vi "Keithley 622x Set DCon.vi"(6 "Step":dbl=0.0001 format="%#_6p", 7 "Delta":dbl=0.0001 format="%#_6p", 8 "error in":errorcluster, 9 "End":dbl=0.001 format="%#_6p", 10 "Start":dbl=-0.001 format="%#_6p", 11 "VISA resource name":refnum<visa-resource-name>) -> (0 "error out":errorcluster, 3 "VISA resource name out":refnum<visa-resource-name>)   [LabVIEW 2021]
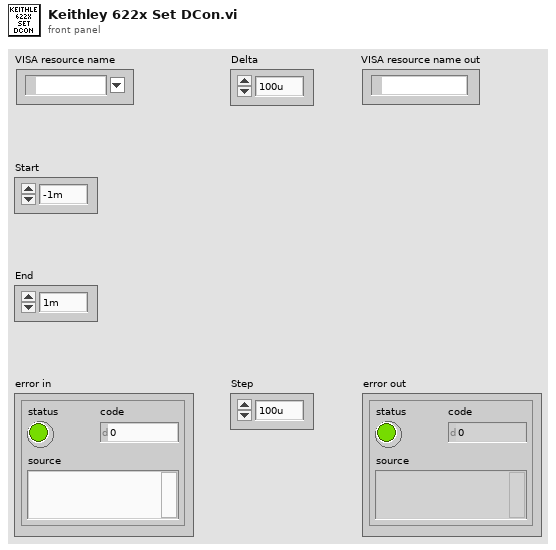
[diagram p1: front panel]
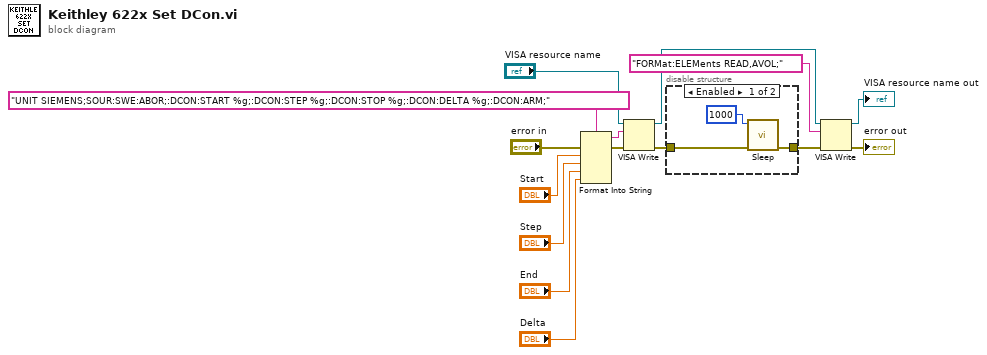
[diagram p0: block diagram]
diagram:
  n1 = Format Into String(format string="UNIT SIEMENS;SOUR:SWE:ABOR;:DCON:START %g;:DCON:STEP %g;:DCON:STOP %g;:DCON:DELTA %g;:DCON:ARM;", error in="error in", "Start", "Step", "End", "Delta") -> (resulting string=w14:string, error out=w15:errorcluster)  [unwired: 1 in]
  n2 = VISA Write(VISA resource name="VISA resource name", write buffer=w14, error in (no error)=w15) -> (VISA resource name out=w13:refnum<visa-resource-name>, error out=w11:errorcluster)  [unwired: 1 out]
  n3 = disable-structure shown="Enabled" {
    disable-tunnel: [w18 w19] -> w10
    disable-tunnel: w11 -> [w16 w19]
    frame Enabled {
      n4 = call "Sleep.vi"("error in"=w16, "milliseconds to wait"=u32 1000) -> ("error out"=w18:errorcluster)  [unwired: 9 in]
    }
    frame Disabled {
    }
  }
  n5 = VISA Write(VISA resource name=w13, write buffer="FORMat:ELEMents READ,AVOL;", error in (no error)=w10) -> (VISA resource name out=→"VISA resource name out":refnum<visa-resource-name>, error out=→"error out":errorcluster)  [unwired: 1 out]
